vi "Persistence Status Value.vi"(1 "Persistence Status In":string, 2 "Read/Write this vi":bool) -> (0 "Persistence Status Out":string)   [LabVIEW 2019]
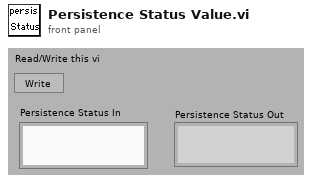
[diagram p1: front panel]
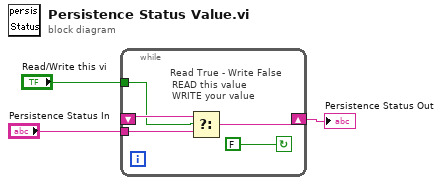
[diagram p0: block diagram]
diagram:
  n1 = while {
    tunnel: "Read/Write this vi" -> [w4]
    shift-right: [w6] -> w1
    shift-left: _ -> [w5]
    tunnel: "Persistence Status In" -> [w7]
    stop <- FALSE continue-if-true
    # "READ this value\nWRITE your value"
    # "Read True - Write False"
    n2 = Select(t=w5, s=w4, f=w7) -> (s? t:f=w6:string)
  }
  "Persistence Status Out" <- w1
